vi "Startup (Event type).vi"(8 "error in (no error)":errorcluster, 11 "Startup Message":refnum<class "MSG.lvclass">) -> (0 "error out":errorcluster, 2 "Command Messenger out":refnum<class "EventMessenger.lvclass">, 3 "Starup Message":refnum<class "MSG.lvclass">)   [LabVIEW 2011, in "Messenging.lvlib" / "Parallel Process.lvclass"]
uses:
  Parallel Process.lvclass
  Interprocess Messenger/TextVarientMessage/MSG.lvclass
  Interprocess Messenger/TextVarientMessage/Reply (message).vi
  Interprocess Messenger/QueueMessenger/QueueMessenger.lvclass
  Interprocess Messenger/EventMessenger/EventMessenger.lvclass
  Interprocess Messenger/LinkedEventMessenger/LinkedEventMessenger.lvclass
  Interprocess Messenger/Messenger (Parent)/MGR.lvclass
  Interprocess Messenger/TextVarientMessage/Write (no data).vi
  Interprocess Messenger/TextVarientMessage/Extract Object (static).vi
  Interprocess Messenger/TextVarientMessage/Write VarMessage.vi
  Interprocess Messenger/VarMessage/VarMessage.lvclass
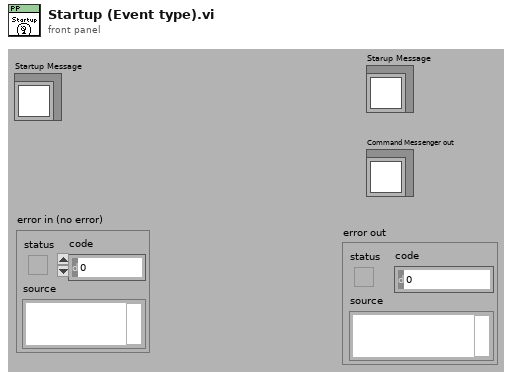
[diagram p1: front panel]
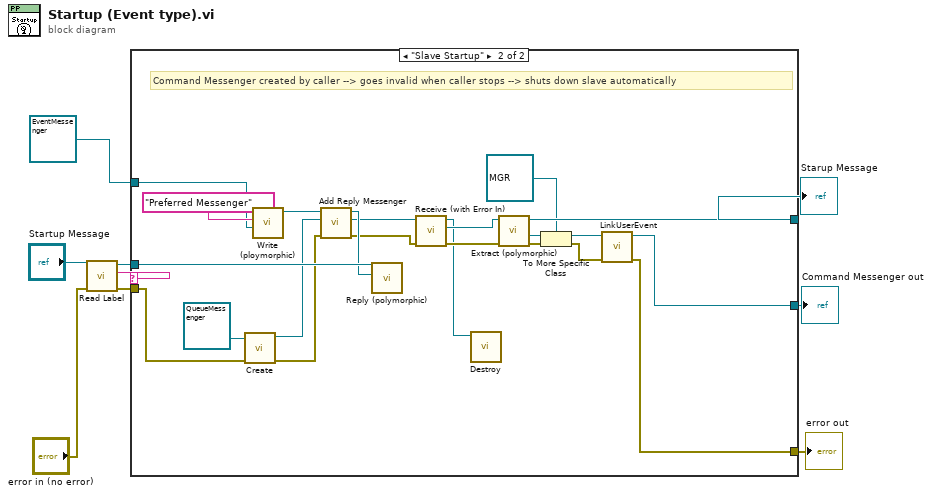
[diagram p0: block diagram]
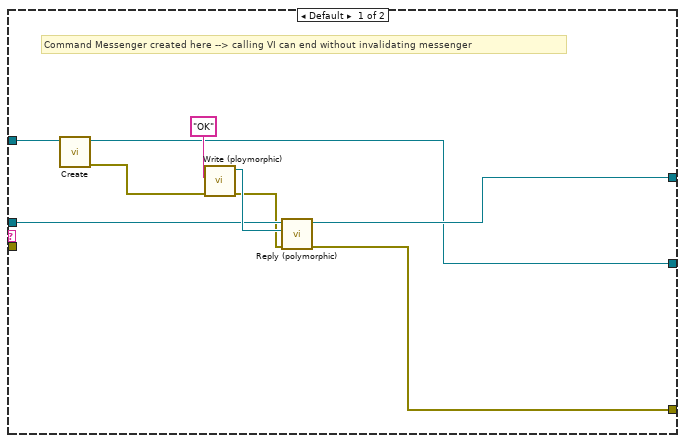
[diagram p2: hidden frame]
diagram:
  n1 = call-dynamic "Read Label.vi"("error in (no error)"="error in (no error)", "Message"="Startup Message") -> ("error out"=w2:errorcluster, "Label"=w8:string, "Message"=w7:refnum<class "MSG.lvclass">)  [unwired: 7 out]
  n2 = case shown="\"Slave Startup\"" w8 {
    tunnel: w7 -> [w15 w38]
    tunnel: refnum<class "EventMessenger.lvclass"> refnum ("Messenging.lvlib:Event Messenger") -> [w18 w34]
    tunnel: [w14 w32] -> w4
    tunnel: [w13 w26] -> w5
    tunnel: w2 -> [_ w20]
    tunnel: [w10 w19] -> w1
    frame Default {
      # "Command Messenger created here --> calling VI can end without invalidating messenger"
      n3 = call-dynamic "Create.vi"("EventMessenger in"=w18) -> ("error out"=w12:errorcluster, "EventMessenger out"=w13:refnum<class "EventMessenger.lvclass">)  [unwired: 1 in, 8 out]
      n4 = call-poly "Write (ploymorphic).vi"("error in (no error)"=w12, "Label"="OK") -> ("error out"=w11:errorcluster, "Message"=w16:refnum<class "MSG.lvclass">)  [unwired: 8 out]
      n5 = call-poly "Reply (polymorphic).vi"("error in (no error)"=w11, "Reply"=w16, "Message to Reply to"=w15) -> ("error out"=w10:errorcluster, "Message"=w14:refnum<class "MSG.lvclass">)  [unwired: 7 out]
    }
    frame "Slave Startup" {
      # "Command Messenger created by caller --> goes invalid when caller stops --> shuts down slave automatically"
      n6 = call-dynamic "Create.vi"("error in (no error)"=w20, "QueueMessenger in"=refnum<class "QueueMessenger.lvclass"> refnum ("QueueMessenger.lvclass")) -> ("error out"=w22:errorcluster, "QueueMessenger out"=w24:refnum<class "QueueMessenger.lvclass">)  [unwired: 8 out]
      n7 = call-poly "Write (ploymorphic).vi"("Varient"=w34, "Label"="Preferred Messenger") -> ("Message"=w39:refnum<class "VarMessage.lvclass">)  [unwired: 1 in, 8 out]
      n8 = call "Add Reply Messenger.vi"("error in (no error)"=w22, "Reply to..."=w24, "Message"=w39) -> ("error out"=w21:errorcluster, "Reply to..."=w36:refnum<class "QueueMessenger.lvclass">, "Message"=w37:refnum<class "VarMessage.lvclass">)  [unwired: 6 out]
      n9 = call-poly "Reply (polymorphic).vi"("Reply"=w37, "Message to Reply to"=w38) -> ()  [unwired: 1 in, 9 out]
      n10 = call-dynamic "Receive (with Error In).vi"("error in (no error)"=w21, "MGR in"=w36) -> ("error out"=w33:errorcluster, "Message"=w35:refnum<class "MSG.lvclass">, "MGR out"=w23:refnum<class "QueueMessenger.lvclass">)  [unwired: 1 in, 6 out]
      n11 = call-dynamic "Destroy.vi"("QueueMessenger in"=w23) -> ()  [unwired: 1 in, 10 out]
      n12 = call-poly "Extract (polymorphic).vi"("error in (no error)"=w33, "ObjMessage in"=w35) -> ("error out"=w31:errorcluster, "Object"=w30:refnum<class>, "ObjMessage out"=w32:refnum<class "MSG.lvclass">)  [unwired: 7 out]
      n13 = To More Specific Class(target class=refnum<class "MGR.lvclass"> refnum ("Messenging.lvlib:MGR.lvclass"), reference=w30, error in=w31) -> (specific class reference=w28:refnum<class "MGR.lvclass">, error out=w27:errorcluster)
      n14 = call "LinkUserEvent.vi"("error in (no error)"=w27, "Messenger in"=w28) -> ("error out"=w19:errorcluster, "EventMessenger out"=w26:refnum<class "EventMessenger.lvclass">)  [unwired: 8 out]
    }
  }
  "Command Messenger out" <- w5
  "Starup Message" <- w4
  "error out" <- w1
